vi "Upgrade Component Dependencies.vi"(0 "NSIS_Installer In":refnum<class "Compound_Installer.lvclass">, 11 "error in (no error)":errorcluster) -> (4 "NSIS_Installer Out":refnum<class "Compound_Installer.lvclass">, 15 "error out":errorcluster)   [LabVIEW 2017, in "CL_G3_VIComponentBuilder.lvlib" / "Compound_Installer.lvclass"]
doc: "Upgrades a component's dependencies. For example, in the case of a VI Package, this VI edits the VIPB to use the latet version of a VI Package's dependencies."
uses:
  Compound_Installer.lvclass
  Exports/Export.lvclass
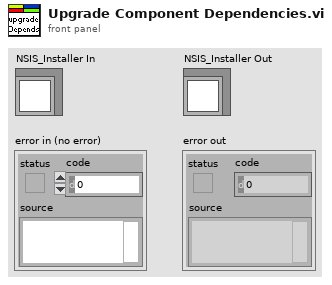
[diagram p1: front panel]
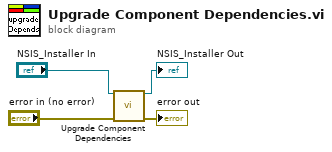
[diagram p0: block diagram]
diagram:
  n1 = call-parent "Upgrade Component Dependencies.vi"("Export In"="NSIS_Installer In", "error in (no error)"="error in (no error)") -> ("Export Out"=→"NSIS_Installer Out":refnum<class "Compound_Installer.lvclass">, "error out"=→"error out":errorcluster)  [unwired: 12 in]
